vi "Longueur d'onde.vi"(11 "T thermistances":dbl[](array[numeric])) -> (3 "Longeur d'onde":dbl)   [LabVIEW 2018]
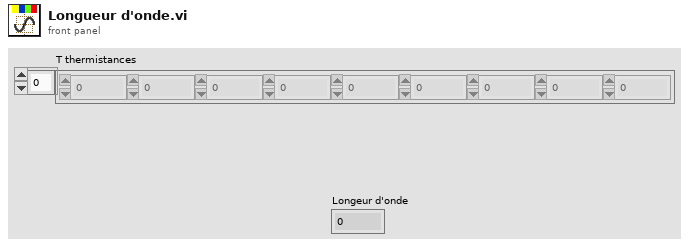
[diagram p1: front panel]
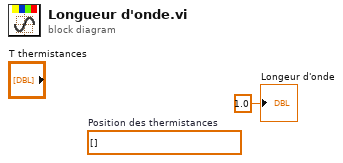
[diagram p0: block diagram]
diagram:
  (unwired) dbl[] []  # Position des thermistances
  "Longeur d'onde" <- 1.0 ("Longeur d'onde")
